vi "DockSubPanelFromFrontPanel.vi"(8 "ErrorIn":errorcluster, 9 "FrontPanel":refnum<class "FrontPanelControl.lvclass">, 10 "PanelLabel":string, 11 "ReferenceIn":refnum<class "MasterGUI.lvclass">) -> (0 "ErrorOut":errorcluster, 3 "ReferenceIn":refnum<class "MasterGUI.lvclass">)   [LabVIEW 2021, in "MasterGUI.lvclass"]
uses:
  MasterGUI.lvclass
  Library_UserInterface_FrontPanelControl/FrontPanelControl/FrontPanelControl.lvclass
  16f1a312-48ec-4227-8a7b-c00f47d308a5.vi
  <vilib>/TriekselSoft/TracerLibrary/TracerLibrary/Tracer/protected/SendMessage.vi
  <vilib>/TriekselSoft/TracerLibrary/TracerLibrary/Tracer/protected/Timestamp.vi
  16f1a312-48ec-4227-8a7b-c00f47d308a5.vi/f75db090-0877-4668-94fb-75c2140b1617.vi
  <vilib>/TriekselSoft/TracerLibrary/TracerLibrary/Tracer/Tracer_Level-Info.vi
  <vilib>/JDP Science/JSONtext/Variant to JSON Text.vi
  <vilib>/TriekselSoft/TracerLibrary/TracerLibrary/Tracer/protected/Tracer_ClassAttributes.vi
  <vilib>/JDP Science/JSONtext/LVClass Serializer/JSONtext LVClass Serializer.lvclass
panel:
  # "s"
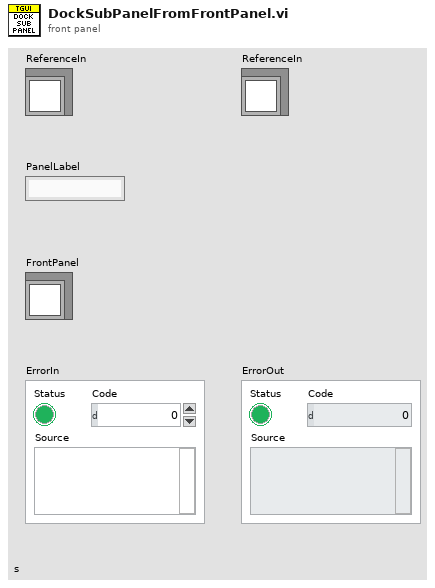
[diagram p1: front panel]
types:
  T1 = typedef "MasterGUI.lvclass/ObjectAttributes.ctl" = cluster{"Interfaces":cluster{"Dummy":refnum<class>}, "Locals":cluster{"MainGUIActive":refnum<queue>, "MainPanel":refnum<vi>, "LayoutPanel":cluster{"PanelVIRef":refnum<vi>, "Labels":string[], "SubPanels":refnum<vi>[]}, "MenuTree":T2[], "Menu":refnum<k9>}, "Persistent":cluster{"StaticDocking":cluster{"ObjectLabel":string, "SubPanelLabel":string}[], "WindowsTitle":string, "AdditionalMenuItems":T2[], "TraceObjectName":string}}
  T2 = typedef "MasterGUI.lvclass/MenuItem.ctl" = cluster{"Parent":string, "Items":string[], "ShortCuts":cluster{"IncludeShiftKey":bool, "IncludeCtrlKey":bool, "ShortcutKey":string}[]}
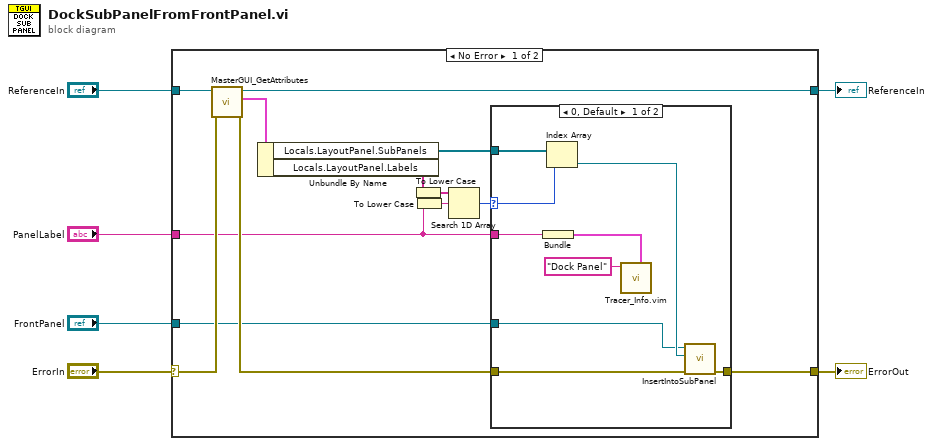
[diagram p0: block diagram]
diagram:
  n1 = case shown="No Error" "ErrorIn" {
    selector: "ErrorIn" -> [w19 w31]
    tunnel: [w17 w31] -> w5
    tunnel: [w14 w30] -> w3
    tunnel: "ReferenceIn" -> [w15 w30]
    tunnel: "PanelLabel" -> [w7 _]
    tunnel: "FrontPanel" -> [w9 _]
    frame No Error {
      n2 = call "MasterGUI_GetAttributes.vi"("ErrorIn"=w19, "ReferenceIn"=w15) -> ("ErrorOut"=w18:errorcluster, "Data"=w16:T1, "ReferenceOut"=w14:refnum<class "MasterGUI.lvclass">)  [unwired: 6 in, 1 out]
      n3 = Unbundle By Name(w16) -> ("Locals.LayoutPanel.SubPanels"=w8:refnum<vi>[], "Locals.LayoutPanel.Labels"=w13:string[])
      n4 = To Lower Case(string=w13) -> (all lower case string=w12:string[])
      n5 = To Lower Case(string=w7) -> (all lower case string=w11:string)
      n6 = Search 1D Array(1D array=w12, element=w11) -> (index of element=w10:i32)  [unwired: 1 in]
      n7 = case shown="0, Default" w10 {
        selector: w10 -> [w25 _]
        tunnel: [w28 w29] -> w17
        tunnel: w18 -> [w27 w29]
        tunnel: w9 -> [w20 _]
        tunnel: w8 -> [w26 _]
        tunnel: w7 -> [w24 _]
        frame 0, Default {
          n8 = Bundle("PanelLabel"=w24) -> (w23:cluster{"PanelLabel":string})  [unwired: 1 in]
          n9 = Index Array(array=w26, index=w25) -> (element=w21:refnum<vi>)
          n10 = call "Tracer_Info.vim"("Data"=w23, "Info Text"="Dock Panel" ("InfoText")) -> ()  [unwired: 9 in, 1 out]
          n11 = call-dynamic "InsertIntoSubPanel.vi"("ErrorIn"=w27, "SubPanelIn"=w21, "ObjectIn"=w20) -> ("ErrorOut"=w28:errorcluster)  [unwired: 7 in, 1 out]
        }
        frame -1 {
        }
      }
    }
    frame Error {
    }
  }
  "ErrorOut" <- w5
  "ReferenceIn" <- w3
